vi "GD_GWID3_F.vi"(8 "error in (no error)":errorcluster, 10 "evaluation_1":i16=1, 11 "DBlink":string="Driver={ODBC Driver 17 for SQL Server};Server=localhost\\SQLEXPRESS;Database=ZDX201;UID=labview;PWD=Dsa@54137926") -> (0 "error out":errorcluster)   [LabVIEW 2019]
uses:
  <vilib>/addons/database/Connection.llb/DB Tools Open Connec (String).vi
  <vilib>/addons/database/Connection.llb/Conn Execute.vi
  <vilib>/addons/database/Recordset.llb/Rec Fetch Recordset Data (R).vi
  <vilib>/addons/database/Recordset.llb/Rec Destroy - Connection.vi
  <vilib>/addons/database/_DB Variant To Data/Database Variant To Data.xnode
  <vilib>/addons/database/NI_Database_API.lvlib
panel:
  out "Command 1":string="SELECT TOP (1) [id]      \n FROM [ZDX201].[dbo].[glue_data]\n where glue_workspace_id=4\nand evaluation_1 is null\norder by id desc "
  out "Command 2":string="WHERE [id]=16"
  in  "columns":string[](array[string])=["evaluation_1", "update_time", "eve_finish_1"]
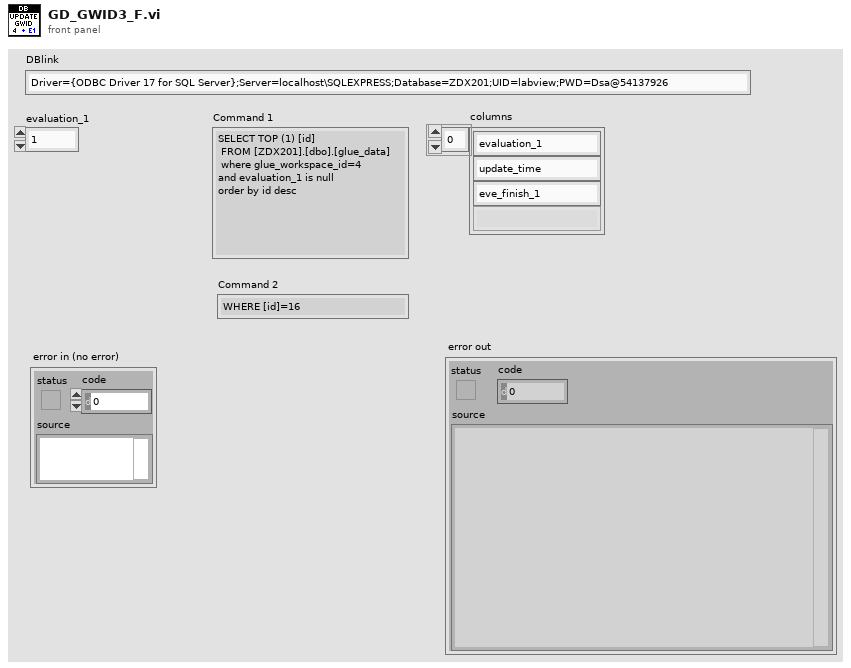
[diagram p1: front panel]
types:
  T1 = cluster{"evaluation_1":string, "update_time":timestamp, "eve_finish_1":timestamp}
  T2 = typedef "NI_Database_API.lvlib/Conn ObjectReference.ctl" = refnum<k1>
  T3 = typedef "NI_Database_API.lvlib/Rec ObjectReference.ctl" = refnum<k1>
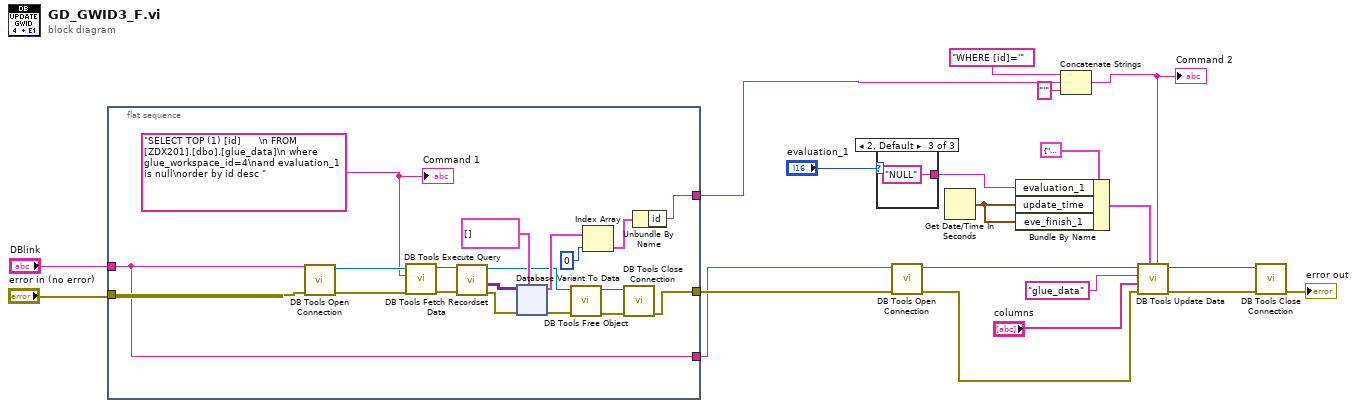
[diagram p0: block diagram]
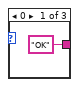
[diagram p2: hidden frame]
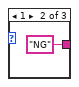
[diagram p3: hidden frame]
diagram:
  n1 = flat-sequence {
    tunnel: "DBlink" -> [w25]
    tunnel: "error in (no error)" -> [w39]
    tunnel: [w26] -> w9
    tunnel: [w25] -> w8
    tunnel: [w22] -> w1
    frame #0 {
      w21 = "SELECT TOP (1) [id]      \n FROM [ZDX201].[dbo].[glue_data]\n where glue_workspace_id=4\nand evaluation_1 is null\norder by id desc " ("SQL query")
      n2 = call-poly <vilib>:"DB Tools Open Connection.vi"("error in (no error)"=w39, "connection information"=w25) -> ("error out"=w38:errorcluster, "connection reference"=w37:T2)  [unwired: 6 in]
      n3 = call-poly <vilib>:"DB Tools Execute Query.vi"("error in (no error)"=w38, "SQL query"=w21, "connection reference"=w37) -> ("error out"=w36:errorcluster, "recordset reference"=w35:T3)  [unwired: 5 in]
      n4 = call-poly <vilib>:"DB Tools Fetch Recordset Data.vi"("error in (no error)"=w36, "recordset reference"=w35) -> ("error out"=w34:errorcluster, "recordset data"=w24:variant[][], "recordset reference out"=w27:T3)  [unwired: 3 in]
      n5 = xnode "Database Variant To Data"("database variant"=w24, "error in (no error)"=w34, "type"=cluster{"id":string}[] [] ("initialized array")) -> ("data"=w32:cluster{"id":string}[], "error out"=w28:errorcluster)
      n6 = call-poly <vilib>:"DB Tools Free Object.vi"("error in (no error)"=w28, "recordset reference"=w27) -> ("error out"=w29:errorcluster, "connection reference"=w30:T2)  [unwired: 8 in]
      n7 = Index Array(array=w32, index=0) -> (element=w23:cluster{"id":string})
      n8 = call <vilib>:"DB Tools Close Connection.vi"("error in (no error)"=w29, "connection reference"=w30) -> ("error out"=w26:errorcluster)  [unwired: 5 in]
      n9 = Unbundle By Name(w23) -> ("id"=w22:string)
      "Command 1" <- w21
    }
  }
  n10 = case shown="2, Default" "evaluation_1" {
    tunnel: ["OK" "NG" "NULL"] -> w5
    frame 0 {
    }
    frame 1 {
    }
    frame 2, Default {
    }
  }
  n11 = call-poly <vilib>:"DB Tools Open Connection.vi"("error in (no error)"=w9, "connection information"=w8) -> ("error out"=w19:errorcluster, "connection reference"=w12:T2)  [unwired: 6 in]
  n12 = Get Date/Time In Seconds() -> (seconds since 1Jan1904=w7:timestamp)
  n13 = Bundle By Name(cluster=T1 {"evaluation_1"="", "update_time"=timestamp(0 s since 1904-01-01), "eve_finish_1"=timestamp(0 s since 1904-01-01)}, "evaluation_1"=w5, "update_time"=w7, "eve_finish_1"=w7) -> (w13:T1)
  n14 = Concatenate Strings("WHERE [id]='", w1, "'" ("string")) -> (w2:string)
  "Command 2" <- w2
  n15 = call <vilib>:"DB Tools Update Data.vi"("condition"=w2, "data"=w13, "error in (no error)"=w19, "columns"="columns", "table"="glue_data", "connection reference"=w12) -> ("error out"=w20:errorcluster, "connection reference out"=w18:T2)  [unwired: 4 in]
  n16 = call <vilib>:"DB Tools Close Connection.vi"("error in (no error)"=w20, "connection reference"=w18) -> ("error out"=→"error out":errorcluster)  [unwired: 5 in]
